vi "FTW-Connector-Close.vi"(0 "FTW Actor Connector":refnum<class "FTW-Actor-Connector.lvclass">, 11 "error in":errorcluster) -> (15 "error out":errorcluster)   [LabVIEW 2013, in "FTW-Actor-Connector.lvclass"]
uses:
  FTW-Actor-Connector.lvclass
  FTW-Actor-Connector.lvclass/FTW-Actor-Connector.ctl
  socket/FTW-Socket.lvclass
panel:
  # "Inputs"
  # "Outputs"
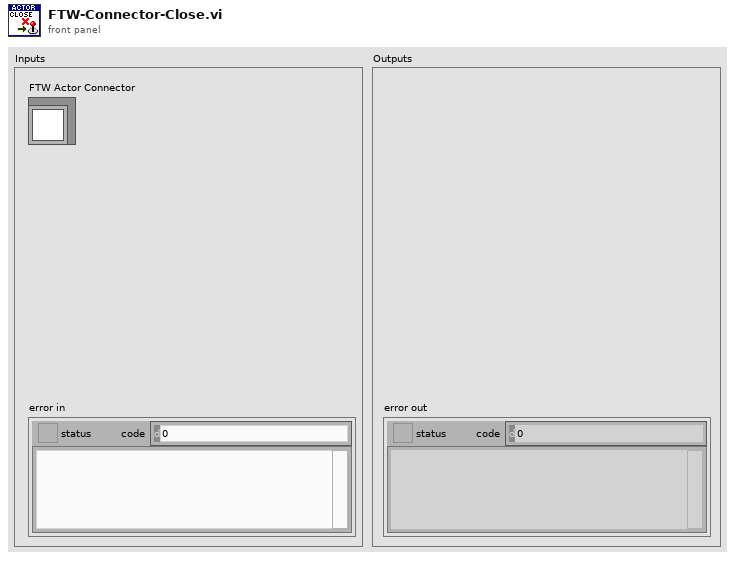
[diagram p1: front panel]
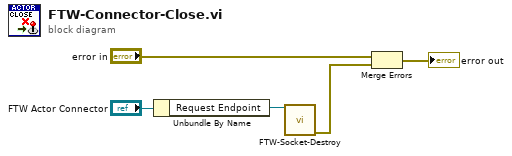
[diagram p0: block diagram]
diagram:
  n1 = Unbundle By Name("FTW Actor Connector") -> ("Request Endpoint"=w2:refnum<class "FTW-Socket.lvclass">)
  n2 = call-dynamic "FTW-Socket-Destroy.vi"("FTW Socket"=w2) -> ("error out"=w1:errorcluster)  [unwired: 14 in]
  n3 = Merge Errors("error in", w1) -> (→"error out":errorcluster)
